vi "NumericSetLimit.vi"(8 "error in":errorcluster, 9 "Control Value":variant, 10 "Control Label":string, 11 "UI Ref cluster in":T1) -> (0 "error out":errorcluster, 3 "UI Ref cluster out":T1)   [LabVIEW 2025, in "UI_Library.lvlib" / "UI_Library.lvclass"]
doc: "Set Numeric Control limit value"
uses:
  UI_Library.lvclass
  Controls/UI_RefCluster.ctl
  <vilib>/Utility/Data Type/Type Definitions/Data Type.ctl
  UI_Library.lvlib
  <vilib>/Utility/Data Type/NI_Data Type.lvlib
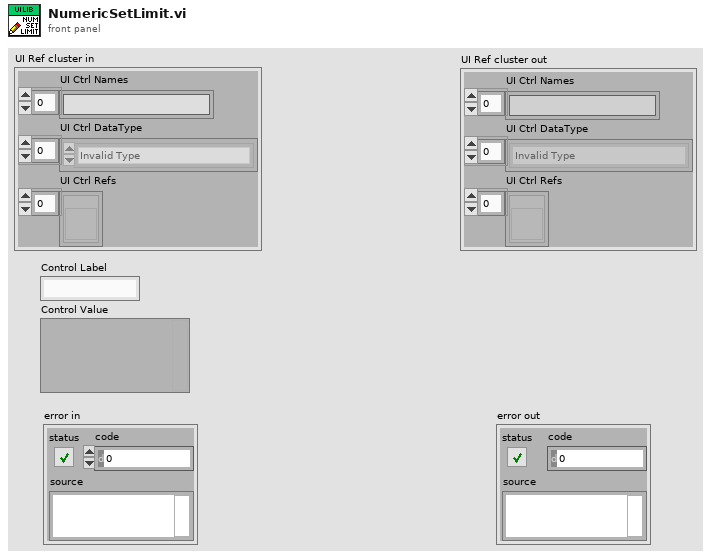
[diagram p1: front panel]
types:
  T1 = typedef "UI_Library.lvlib/UI_RefCluster.ctl" = cluster{"UI Ctrl Names":string[], "UI Ctrl DataType":T2[], "UI Ctrl Refs":refnum<vi>[]}
  T2 = typedef "NI_Data Type.lvlib/Data Type.ctl" = enum8{"Invalid Type", "Void", "I8", "I16", "I32", "I64", "U8", "U16", "U32", "U64", "Single Float", "Double Float", "Extended Float", "Single Complex", "Double Complex", "Extended Complex", "Enum U8", "Enum U16", "Enum U32", "Enum U64", "Single Float With Unit", "Double Float With Unit", "Extended Float With Unit", "Single Complex with Unit", "Double Complex with Unit", "Extended Complex with Unit", "Boolean", "String", "Path", "Picture", "Tag", "Array", "Cluster", "Variant", "LV Variant", "Waveform", "Timestamp", "Digital Waveform", "Digital Data", "ExpressData", "Refnum", "External Data", "VI", "Poly VI", "LabVIEW Class Instance", "Fixed Point", "Set Collection", "Map Collection"}
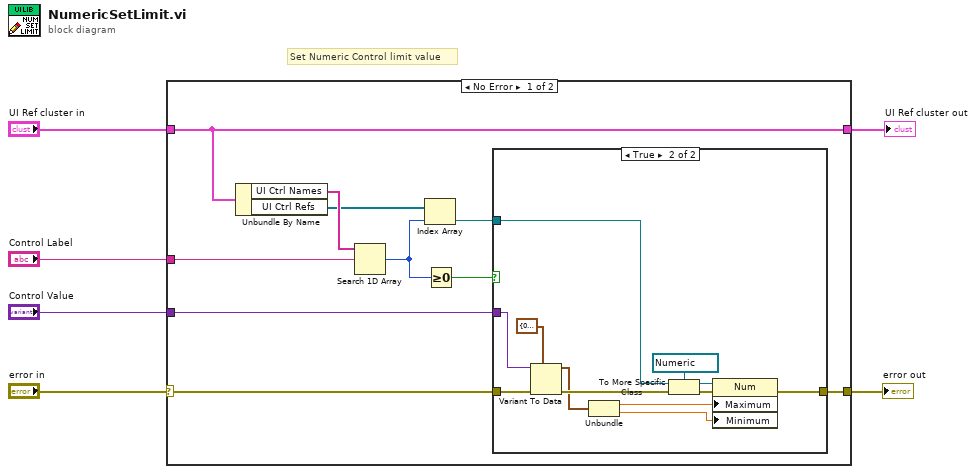
[diagram p0: block diagram]
diagram:
  # "Set Numeric Control limit value"
  n1 = case shown="No Error" "error in" {
    selector: "error in" -> [w11 w31]
    tunnel: [w10 w31] -> w6
    tunnel: "Control Value" -> [w9 _]
    tunnel: "Control Label" -> [w15 _]
    tunnel: [w8 w30] -> w2
    tunnel: "UI Ref cluster in" -> [w8 w30]
    frame No Error {
      n2 = Unbundle By Name(w8) -> ("UI Ctrl Names"=w16:string[], "UI Ctrl Refs"=w14:refnum<vi>[])
      n3 = Search 1D Array(1D array=w16, element=w15) -> (index of element=w13:i32)  [unwired: 1 in]
      n4 = Index Array(array=w14, index=w13) -> (element=w12:refnum<vi>)
      n5 = Greater Or Equal To 0?(x=w13) -> (x >= 0?=w7:bool)
      n6 = case shown="True" w7 {
        tunnel: w12 -> [_ w22]
        tunnel: w11 -> [w17 w26]
        tunnel: [w17 w23] -> w10
        tunnel: w9 -> [_ w25]
        frame False {
        }
        frame True {
          n7 = Variant To Data(error in=w26, type=cluster{"Maximum":dbl, "Minimum":dbl} {"Maximum"=0.0, "Minimum"=0.0}, Variant=w25) -> (data=w20:cluster{"Maximum":dbl, "Minimum":dbl}, error out=w24:errorcluster)
          n8 = Unbundle(w20) -> ("Maximum"=w19:dbl, "Minimum"=w18:dbl)
          n9 = To More Specific Class(target class=refnum<vi> refnum ("reference"), reference=w22, error in=w24) -> (specific class reference=w27:refnum<vi>, error out=w29:errorcluster)
          n10 = property class="Num"(reference=w27, error in=w29, "Maximum"=w19, "Minimum"=w18) -> (error out=w23:errorcluster)  [unwired: 1 out]
        }
      }
    }
    frame Error {
    }
  }
  "error out" <- w6
  "UI Ref cluster out" <- w2
